vi "MGSE Append Log.vi"(11 "Log Line":string) -> (3 "log dup":string)   [LabVIEW 2018]
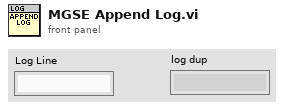
[diagram p1: front panel]
types:
  T1 = enum16{"open", "replace", "create", "open or create", "replace or create", "replace or create with confirmation"}
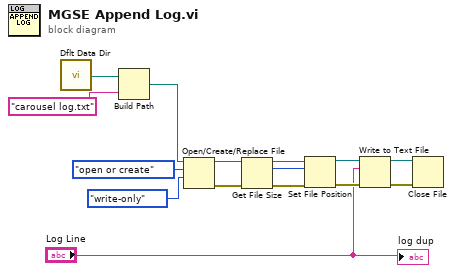
[diagram p0: block diagram]
diagram:
  n1 = call <vilib>:"Dflt Data Dir.vi"() -> ("App:Default Data Directory"=w15:path)
  n2 = Build Path(base path=w15, name or relative path="carousel log.txt") -> (appended path=w13:path)
  n3 = Open/Create/Replace File(file path (use dialog)=w13, operation (0:open)=T1."open or create", access (0:read/write)=enum16{"read/write", "read-only", "write-only"}."write-only") -> (refnum out=w9:refnum<file>, error out=w10:errorcluster)  [unwired: 3 in, 1 out]
  n4 = Get File Size(file=w9, error in=w10) -> (refnum out=w8:refnum<file>, size (in bytes)=w7:i64, 0:w6:errorcluster)
  n5 = Set File Position(offset (in bytes) (0)=w7, refnum=w8, error in=w6) -> (refnum out=w4:refnum<file>, error out=w5:errorcluster)  [unwired: 1 in]
  n6 = Write to Text File(file (use dialog)=w4, text="Log Line", error in=w5) -> (refnum out=w1:refnum<file>, error out=w2:errorcluster)  [unwired: 1 in, 1 out]
  n7 = Close File(refnum=w1, error in=w2) -> ()  [unwired: 2 out]
  "log dup" <- "Log Line"
